vi "Motor Control_ angle conversion.vi"(2 "Motor Speed":dbl(slide)=10.0 scale=-10.0..10.0, 3 "reference angle":dbl=59.85 format="%#_13g", 4 "Reset motor counts":bool, 5 "target angle":dbl=55.0 format="%#_13g") -> (1 "actual angle":dbl=54.999976091263065)   [LabVIEW 2015]
uses:
  <vilib>/Analysis/1siggen.llb/Ramp Pattern by Samples.vi
  <vilib>/DAQmx/write.llb/DAQmx Write (Analog 1D DBL 1Chan NSamp).vi
  <vilib>/DAQmx/read.llb/DAQmx Read (Counter U32 1Chan 1Samp).vi
  <vilib>/DAQmx/create/channels.llb/DAQmx Create Channel (CI-Position-Angular Encoder).vi
  <vilib>/DAQmx/create/channels.llb/DAQmx Create Channel (AO-Voltage-Basic).vi
  <vilib>/DAQmx/configure/timing.llb/DAQmx Timing (Sample Clock).vi
  <vilib>/DAQmx/miscellaneous.llb/DAQmx Fill In Error Info.vi
  Global Variable.vi
  <resource>/objmgr/daqmx.rc
  <vilib>/ptbypt/NI_PtbyPt.lvlib
  <vilib>/Analysis/NI_AALBase.lvlib
panel:
  out "Numeric":i32=23554
  out "error out":errorcluster={"status"=TRUE, "code"=-200288, "source"="Motor Control_ angle conversion.vi<append>\n<B>Attempted to Write Sample: </B>1000\n<B>Property: </B>RelativeTo\n<B>Corresponding Value: </B>Current Write Position\n<B>Property: </B>Offset\n<B>Corresponding Value: </B>0\n\n<B>Task Name: </B>_unnamedTask<9>"}
  out "Indicator of current\n motor pulse":i32=141999
  out "Waveform Chart":i32(graph)=141999
  out "Target  Pulse":dbl=141998.3000000001
  out "Motor Pulses":i32=141999
  in  "stop":bool
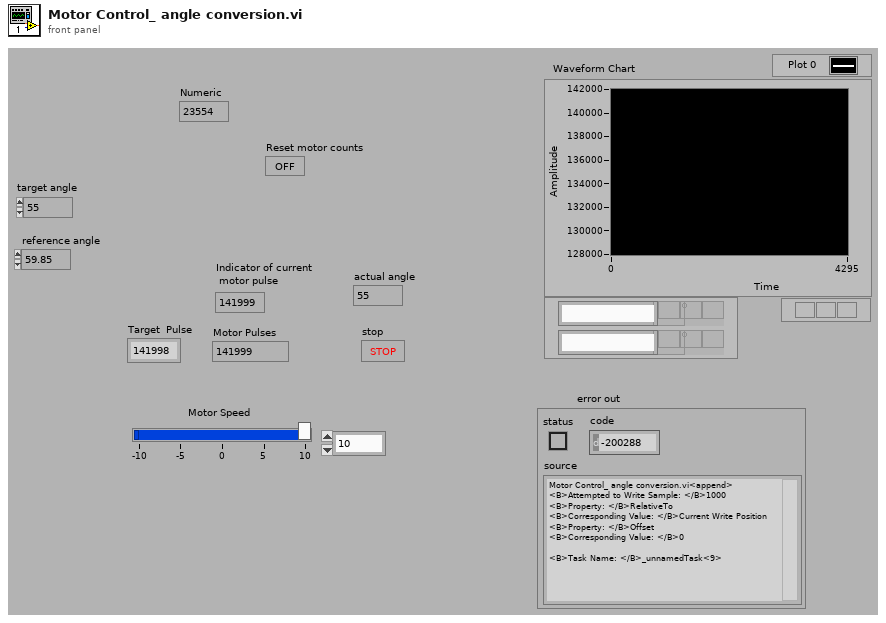
[diagram p1: front panel]
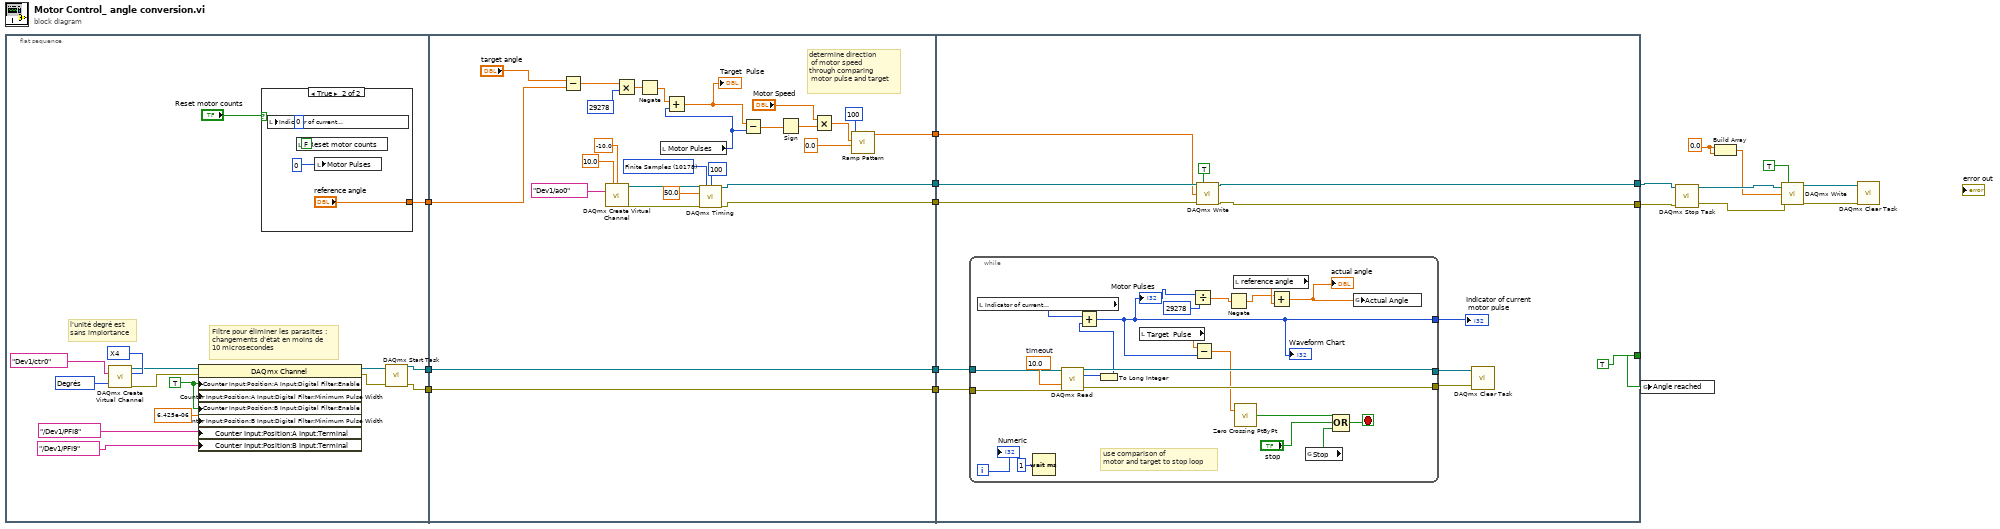
[diagram p0: block diagram]
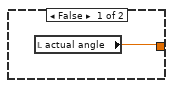
[diagram p2: hidden frame]
diagram:
  w2 = 0.0 ("data")
  n1 = flat-sequence {
    tunnel: [w32] -> w13
    tunnel: [w20] -> w12
    tunnel: [w19] -> w11
    tunnel: [w51] -> w16
    tunnel: [w50] -> w15
    tunnel: w13 -> [w52]
    tunnel: w12 -> [w51]
    tunnel: w11 -> [w50]
    tunnel: [w42] -> w10
    tunnel: [w41] -> w9
    tunnel: [w40] -> w8
    tunnel: w16 -> [w74]
    tunnel: w15 -> [w73]
    tunnel: [w69] -> w5
    tunnel: [TRUE] -> w14
    tunnel: w10 -> [w71]
    tunnel: w9 -> [w70]
    tunnel: [w68] -> w6
    tunnel: w8 -> [w67]
    frame #0 {
      w26 = 10146 items=["Degrés"=10146, "Radians"=10273, "Tops"=10304, "À partir d'une échelle personnalisée"=10065] ("units")
      w25 = 10092 items=["X1"=10090, "X2"=10091, "X4"=10092, "Comptage de deux impulsions"=10313] ("decoding type")
      w21 = 6.425e-06 ("CI.Encodeur.EntréeA.FltrNum.LargImpMin")
      w22 = TRUE ("CI.Encodeur.Entrée.FltrNum.Activer")
      # "l'unité degré est\nsans impiortance"
      # "Filtre pour éliminer les parasites :\nchangements d'état en moins de\n10 microsecondes"
      n2 = call-poly <vilib>:"DAQmx Create Virtual Channel.vi"("counter"=tag "Dev1/ctr0", "decoding type"=w25, "units"=w26) -> ("task out"=w23:refnum<k21>, "error out"=w24:errorcluster)  [unwired: 11 in]
      n3 = property class="DAQmx Channel"(reference=w23, error in=w24, "Counter Input:Position:A Input:Digital Filter:Enable"=w22, "Counter Input:Position:A Input:Digital Filter:Minimum Pulse Width"=w21, "Counter Input:Position:B Input:Digital Filter:Enable"=w22, "Counter Input:Position:B Input:Digital Filter:Minimum Pulse Width"=w21, "Counter Input:Position:A Input:Terminal"=tag "/Dev1/PFI8" ("CI.Encodeur.TermEntréeB"), "Counter Input:Position:B Input:Terminal"=tag "/Dev1/PFI9" ("CI.Encodeur.TermEntréeB")) -> (reference out=w30:refnum<k21>, error out=w31:errorcluster)
      n4 = case shown="True" "Reset motor counts" {
        tunnel: [w34 "reference angle"] -> w32
        frame False {
          n5 = local read "actual angle"() -> (w34:dbl)
        }
        frame True {
          n6 = local write "Indicator of current\n motor pulse"(0 ("Numeric 2")) -> ()
          n7 = local write "Reset motor counts"(FALSE ("Boolean")) -> ()
          n8 = local write "Motor Pulses"(0 ("Motor Pulses")) -> ()
        }
      }
      n9 = call <vilib>:"DAQmx Start Task.vi"("task/channels in"=w30, "error in"=w31) -> ("task out"=w20:refnum<k21>, "error out"=w19:errorcluster)  [unwired: 12 in]
    }
    frame #1 {
      w43 = 10178 items=["Finite Samples"=10178, "Continuous Samples"=10123, "Hardware Timed Single Point"=12522] ("sample mode")
      # "determine direction\n of motor speed\nthrough comparing\n motor pulse and target"
      n10 = Subtract(x="target angle", y=w52) -> (x-y=w57:dbl)
      n11 = call-poly <vilib>:"DAQmx Create Virtual Channel.vi"("maximum value"=10.0, "minimum value"=-10.0, "physical channels"=tag "Dev1/ao0") -> ("task out"=w46:refnum<k21>, "error out"=w45:errorcluster)  [unwired: 11 in]
      n12 = Multiply(x=w57, y=29278) -> (x*y=w56:dbl)
      n13 = Negate(x=w56) -> (-x=w55:dbl)
      n14 = local read "Motor Pulses"() -> (w53:i32)
      n15 = Add(x=w55, y=w53) -> (x+y=w54:dbl)
      "Target  Pulse" <- w54
      n16 = call-poly <vilib>:"DAQmx Timing.vi"("task/channels in"=w46, "sample mode"=w43, "samples per channel"=100, "rate"=50.0, "error in"=w45) -> ("task out"=w42:refnum<k21>, "error out"=w41:errorcluster)  [unwired: 9 in]
      n17 = Subtract(x=w54, y=w53) -> (x-y=w61:dbl)
      n18 = Sign(1:w61) -> (0:w62:dbl)
      n19 = Multiply(x="Motor Speed", y=w62) -> (x*y=w49:dbl)
      n20 = call-poly <vilib>:"Ramp Pattern.vi"("start"=0.0, "end"=w49, "samples"=100) -> ("Ramp Pattern"=w40:dbl[])  [unwired: 7 in, 1 out]
    }
    frame #2 {
      n21 = while {
        tunnel: [w96] -> w76
        tunnel: [w95] -> w75
        tunnel: [w85] -> w77
        tunnel: w74 -> [w90]
        tunnel: w73 -> [w89]
        i -> [w79]
        stop <- w94 stop-if-true
        w97 = 10.0  # timeout
        # "use comparison of\nmotor and target to stop loop"
        n22 = local read "Indicator of current\n motor pulse"() -> (w92:i32)
        n23 = Wait (ms)(milliseconds to wait=u32 1 ("attente (ms)")) -> ()  [unwired: 1 out]
        n24 = call-poly <vilib>:"DAQmx Read.vi"("task/channels in"=w90, "timeout"=w97, "error in"=w89) -> ("task out"=w96:refnum<k21>, "data"=w98:u32, "error out"=w95:errorcluster)  [unwired: 10 in]
        n25 = To Long Integer(number=w98) -> (32bit integer=w91:i32)
        n26 = Add(x=w92, y=w91) -> (x+y=w85:i32)
        "Waveform Chart" <- w85
        "Motor Pulses" <- w85
        n27 = local read "Target  Pulse"() -> (w88:dbl)
        n28 = Divide(x=w85, y=29278) -> (x/y=w82:dbl)
        n29 = Subtract(x=w88, y=w85) -> (x-y=w87:dbl)
        n30 = Negate(x=w82) -> (-x=w81:dbl)
        n31 = local read "reference angle"() -> (w83:dbl)
        n32 = call <vilib>:"Zero Crossing PtByPt.vi"("input data point"=w87) -> ("crossing"=w86:bool)  [unwired: 2 in]
        n33 = Add(x=w81, y=w83) -> (x+y=w80:dbl)
        "actual angle" <- w80
        n34 = global read "Global Variable.vi" "Stop"() -> (w78:bool)
        n35 = Compound Arithmetic op=OR(w86, "stop", w78) -> (w94:bool)
        n36 = global write "Global Variable.vi" "Actual Angle"(w80) -> ()
        "Numeric" <- w79
      }
      "Indicator of current\n motor pulse" <- w77
      n37 = call-poly <vilib>:"DAQmx Write.vi"("task/channels in"=w71, "auto start"=TRUE, "data"=w67, "error in"=w70) -> ("task out"=w68:refnum<k21>, "error out"=w69:errorcluster)  [unwired: 9 in, 1 out]
      n38 = call <vilib>:"DAQmx Clear Task.vi"("task in"=w76, "error in"=w75) -> ()  [unwired: 13 in, 1 out]
    }
  }
  n39 = global write "Global Variable.vi" "Angle reached"(w14) -> ()
  n40 = call <vilib>:"DAQmx Stop Task.vi"("task/channels in"=w6, "error in"=w5) -> ("task out"=w4:refnum<k21>, "error out"=w3:errorcluster)  [unwired: 12 in]
  n41 = Build Array(w2, w2) -> (w1:dbl[])
  n42 = call-poly <vilib>:"DAQmx Write.vi"("task/channels in"=w4, "auto start"=TRUE, "data"=w1, "error in"=w3) -> ("task out"=w18:refnum<k21>, "error out"=w17:errorcluster)  [unwired: 9 in, 1 out]
  n43 = call <vilib>:"DAQmx Clear Task.vi"("task in"=w18, "error in"=w17) -> ()  [unwired: 13 in, 1 out]
